vi "Initialize Settings.vi"(11 "error in (no error)":errorcluster) -> (6 "VISA resource name 2":refnum<visa-resource-name>, 15 "error out":errorcluster)   [LabVIEW 2013, in "Scale.lvlib" / "Scale.lvclass"]
uses:
  Scale.lvclass
panel:
  in  "Scale COM Port":refnum<visa-resource-name>
  in  "Button":bool
  # "Enter Scale COM Port"
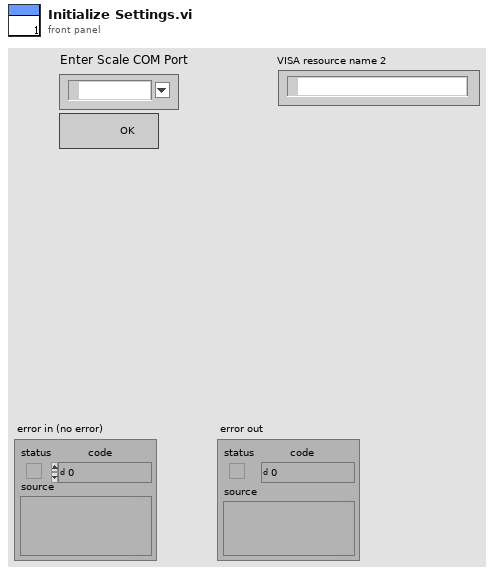
[diagram p1: front panel]
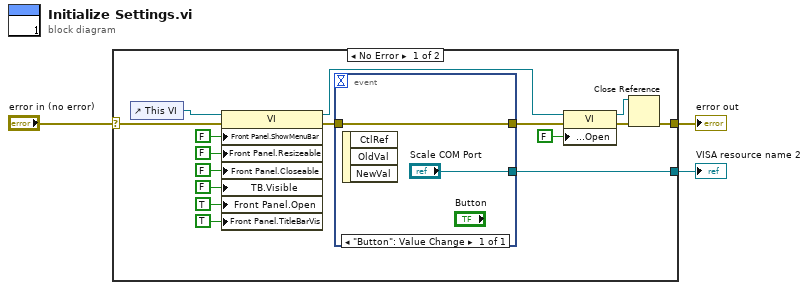
[diagram p0: block diagram]
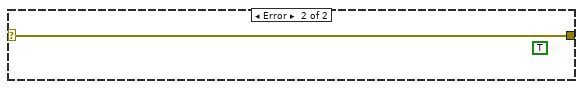
[diagram p2: hidden frame]
diagram:
  n1 = case shown="No Error" "error in (no error)" {
    selector: "error in (no error)" -> [w12 w22]
    tunnel: [w7 w22] -> w2
    tunnel: [w4 _] -> w1
    frame No Error {
      n2 = control-ref of="This VI"() -> (w19:refnum<vi>)
      n3 = property class="VI"(reference=w19, error in=w12, "Front Panel.ShowMenuBar"=FALSE ("Front Panel Window:Show Menu Bar"), "Front Panel.Resizeable"=FALSE ("Front Panel Window:Resizable"), "Front Panel.Closeable"=FALSE ("Front Panel Window:Closeable"), "TB.Visible"=FALSE ("Tool Bar:Visible"), "Front Panel.Open"=TRUE ("Front Panel Window:Open"), "Front Panel.TitleBarVis"=TRUE ("Front Panel Window:Title Bar Visible")) -> (reference out=w6:refnum<vi>, error out=w11:errorcluster)
      n4 = event shown="[0] \"Button\": Value Change" {
        selector: _ -> [_]
        dyn-events: _ -> [_]
        timeout: _ -> [_]
        tunnel: w11 -> [w21]
        tunnel: [w21] -> w5
        tunnel: ["Scale COM Port"] -> w4
        event "Button": Value Change {
          n5 = event-data() -> ()  [unwired: 1 in, 3 out]
        }
      }
      n6 = property class="VI"(reference=w6, error in=w5, "Front Panel.Open"=FALSE ("Front Panel Window:Open")) -> (reference out=w10:refnum<vi>, error out=w9:errorcluster)
      n7 = Close Reference(reference=w10, error in (no error)=w9) -> (error out=w7:errorcluster)
    }
    frame Error {
      (unwired) TRUE ("Front Panel Window:Open")
    }
  }
  "error out" <- w2
  "VISA resource name 2" <- w1
